vi "getNormalTempIndex.vi"(10 "索引温度":dbl=20.0, 11 "温度列表":dbl[](array[numeric])) -> (3 "常温索引":dbl)   [LabVIEW 2017]
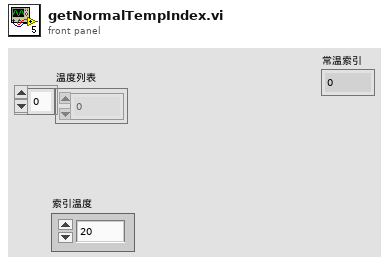
[diagram p1: front panel]
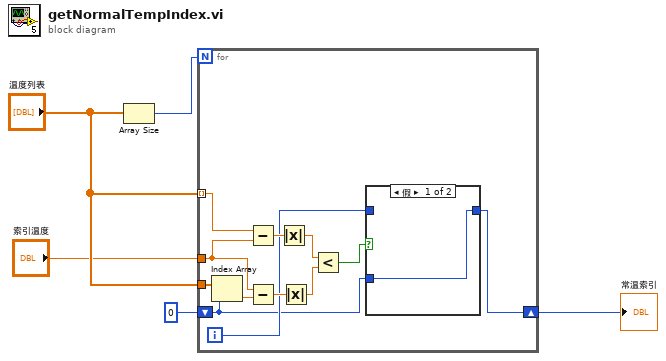
[diagram p0: block diagram]
diagram:
  n1 = Array Size(array="温度列表") -> (size(s)=w5:i32)
  n2 = for {
    N: w5 -> [_]
    tunnel: "温度列表" -> [w12] mode=indexing
    shift-right: [w11] -> w4
    shift-left: 0 ("索引") -> [w8]
    tunnel: "温度列表" -> [w9]
    tunnel: "索引温度" -> [w6]
    i -> [w10]
    n3 = Index Array(array=w9, index=w8) -> (element=w7:dbl)
    n4 = Subtract(x=w12, y=w6) -> (x-y=w17:dbl)
    n5 = Subtract(x=w6, y=w7) -> (x-y=w16:dbl)
    n6 = Absolute Value(x=w17) -> (abs(x)=w15:dbl)
    n7 = Absolute Value(x=w16) -> (abs(x)=w14:dbl)
    n8 = Less?(x=w15, y=w14) -> (x < y?=w13:bool)
    n9 = case shown="假" w13 {
      tunnel: w10 -> [_ w19]
      tunnel: [w18 w19] -> w11
      tunnel: w8 -> [w18 _]
      frame False {
      }
      frame True {
      }
    }
  }
  "常温索引" <- w4
